vi "sql.vi"(2 "SQL query":string, 3 "error in (no error)":errorcluster) -> (0 "error out":errorcluster)   [LabVIEW 2014]
uses:
  <vilib>/addons/database/Connection.llb/DB Tools Open Connec (String).vi
  <vilib>/addons/database/Connection.llb/Conn Execute.vi
  <vilib>/addons/database/Recordset.llb/Rec Fetch Recordset Data (R).vi
  <vilib>/addons/database/Recordset.llb/Rec Destroy - Connection.vi
  <vilib>/addons/database/NI_Database_API.lvlib
panel:
  out "多列列表框":i32(listbox)
  out "结果字符串":string
  # "INSERT INTO  X00037AD  VALUES('AAA','SSSS','CCCC',11,'EEE',3445,22)"
  # "insert into X00037AD \n (DT,ST,SV,SNL,TN,PI,SN  )    values (00123,‘张涛’,'Administrator','张涛.JPG','2018/3/17','D:\\Users\\张涛.JPG',019782)"
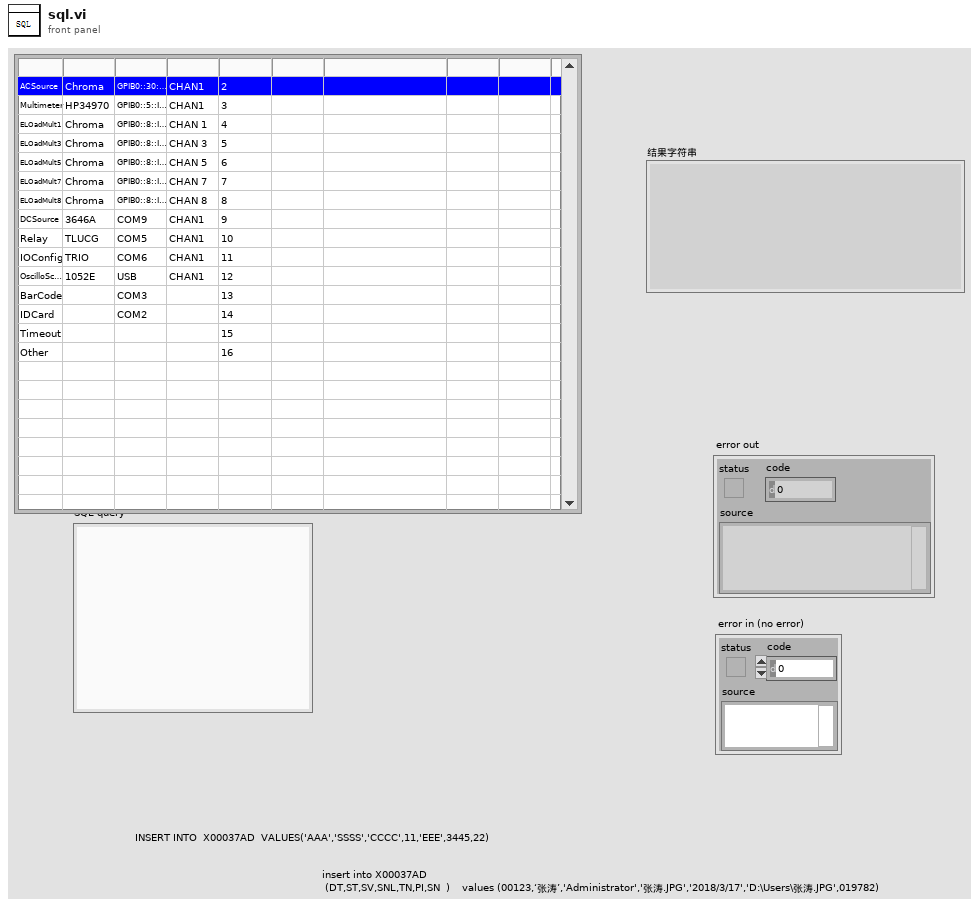
[diagram p1: front panel]
types:
  T1 = typedef "NI_Database_API.lvlib/Conn ObjectReference.ctl" = refnum<k1>
  T2 = typedef "NI_Database_API.lvlib/Rec ObjectReference.ctl" = refnum<k1>
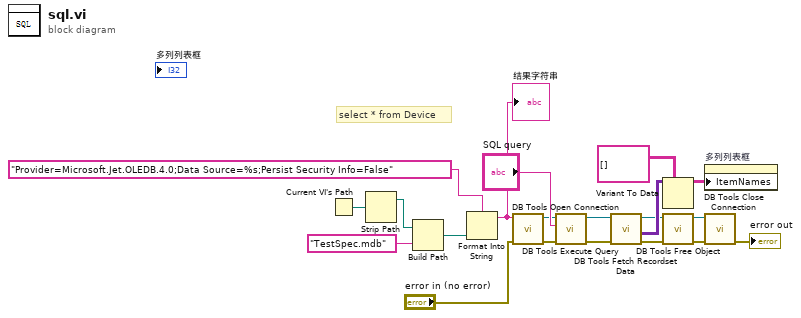
[diagram p0: block diagram]
diagram:
  # "select * from Device"
  n1 = Current VI's Path() -> (path=w7:path)
  n2 = Strip Path(path=w7) -> (stripped path=w6:path)  [unwired: 1 out]
  n3 = Build Path(base path=w6, name or relative path="TestSpec.mdb") -> (appended path=w4:path)
  n4 = Format Into String(format string="Provider=Microsoft.Jet.OLEDB.4.0;Data Source=%s;Persist Security Info=False" ("初始字符串"), w4) -> (resulting string=w1:string)  [unwired: 2 in, 1 out]
  "结果字符串" <- w1
  n5 = call-poly <vilib>:"DB Tools Open Connection.vi"("error in (no error)"="error in (no error)", "connection information"=w1) -> ("error out"=w9:errorcluster, "connection reference"=w14:T1)  [unwired: 6 in]
  n6 = call-poly <vilib>:"DB Tools Execute Query.vi"("error in (no error)"=w9, "SQL query"="SQL query", "connection reference"=w14) -> ("error out"=w8:errorcluster, "recordset reference"=w13:T2)  [unwired: 5 in]
  n7 = call-poly <vilib>:"DB Tools Fetch Recordset Data.vi"("error in (no error)"=w8, "recordset reference"=w13) -> ("error out"=w19:errorcluster, "recordset data"=w16:variant[][], "recordset reference out"=w12:T2)  [unwired: 3 in]
  n8 = Variant To Data(type=string[][] [], Variant=w16) -> (data=w2:string[][])  [unwired: 1 in, 1 out]
  n9 = call-poly <vilib>:"DB Tools Free Object.vi"("error in (no error)"=w19, "recordset reference"=w12) -> ("error out"=w18:errorcluster, "connection reference"=w11:T1)  [unwired: 8 in]
  n10 = property on="多列列表框" class="MCListbox (严格)"("ItemNames"=w2) -> ()  [unwired: 2 in, 2 out]
  n11 = call <vilib>:"DB Tools Close Connection.vi"("error in (no error)"=w18, "connection reference"=w11) -> ("error out"=→"error out":errorcluster)  [unwired: 5 in]
